vi "SLL DE AO Driver.vi"(6 "AO Channel Value Array":dbl[](array[numeric]), 7 "AO Driver Option":T2=enum."Read Full Status", 8 "error in (no error)":errorcluster, 9 "AO Channel Value":dbl, 10 "AO Channel Name Array":T1[](array[typedef]), 11 "AO Channel Name":T1) -> (0 "error out":errorcluster)   [LabVIEW 2013]
doc: "Copyright © 2005, Soliton Technologies.\nAll rights reserved."
uses:
  Controls/SLL DE AO Global Options.ctl
  Controls/SLL DE List of Analog Outputs.ctl
  Controls/SLL DE DAQ Global Options.ctl
  Controls/SLL DE DAQ Global Elements.ctl
  Controls/SLL DE AO Min Max Range Checking Options.ctl
  Controls/SLL DE AO Safe Value Global Options.ctl
  <vilib>/DAQmx/write.llb/DAQmx Write (Analog DBL 1Chan 1Samp).vi
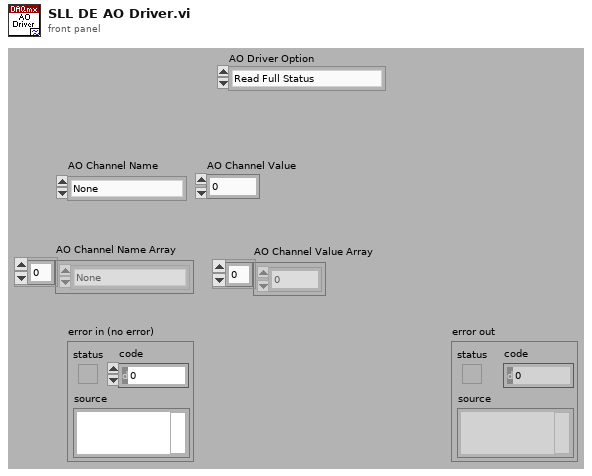
[diagram p1: front panel]
types:
  T1 = typedef "SLL DE List of Analog Outputs.ctl" = enum16{"None"}
  T2 = typedef "SLL DE AO Global Options.ctl" = enum16{"Init", "Write Line", "Write Array", "Read Line", "Read Array", "Read Full Status", "Restart AO", "Send to Safe Mode", "Stop AO"}
  T3 = typedef "SLL DE DAQ Global Elements.ctl" = enum16{"AI Error", "AO Error", "DI Error", "DO Error", "AI Restart", "DI Restart", "AI Running", "AO Running", "DI Running", "DO Running", "DAQ Exit?"}
  T4 = typedef "SLL DE DAQ Global Options.ctl" = enum16{"Init", "Write 1", "Read 1", "Write Array", "Read Array", "Clear"}
  T5 = typedef "SLL DE AO Min Max Range Checking Options.ctl" = enum16{"Initalize Channel Range", "Check Single AO Channel", "Check Multiple AO Channels"}
  T6 = typedef "SLL DE AO Safe Value Global Options.ctl" = enum16{"Read", "Write"}
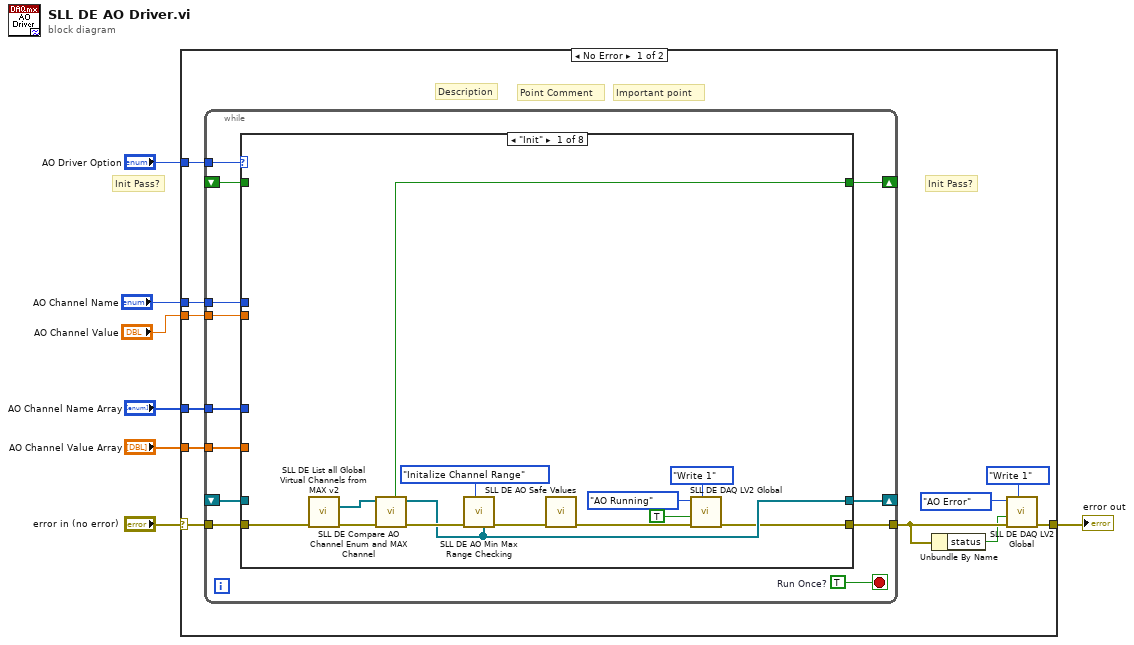
[diagram p0: block diagram]
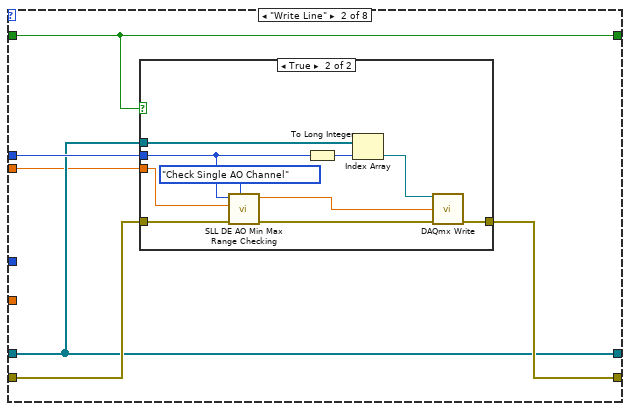
[diagram p2: hidden frame]
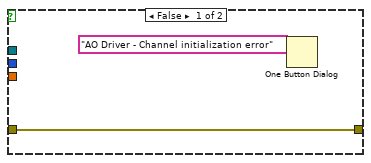
[diagram p3: hidden frame]
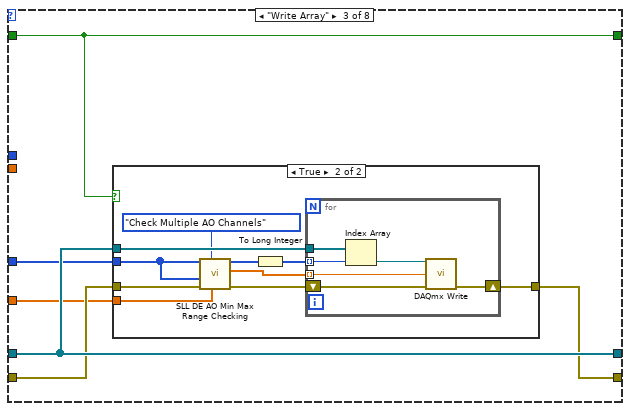
[diagram p4: hidden frame]
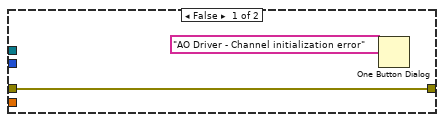
[diagram p5: hidden frame]
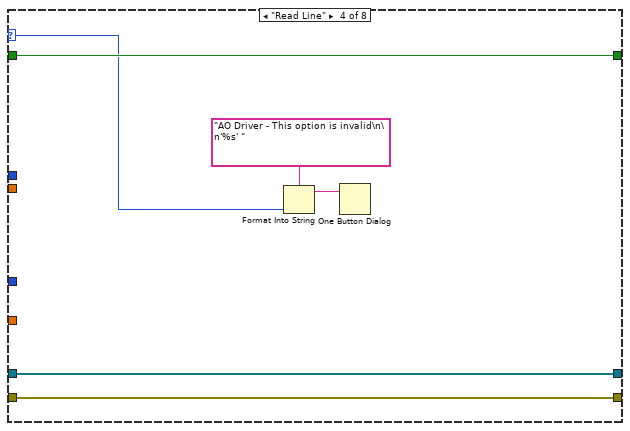
[diagram p6: hidden frame]
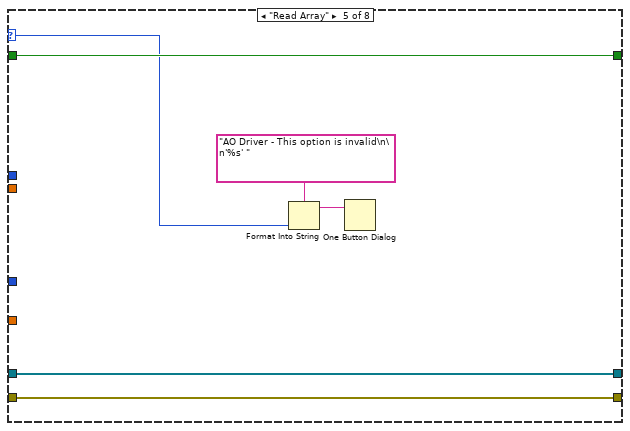
[diagram p7: hidden frame]
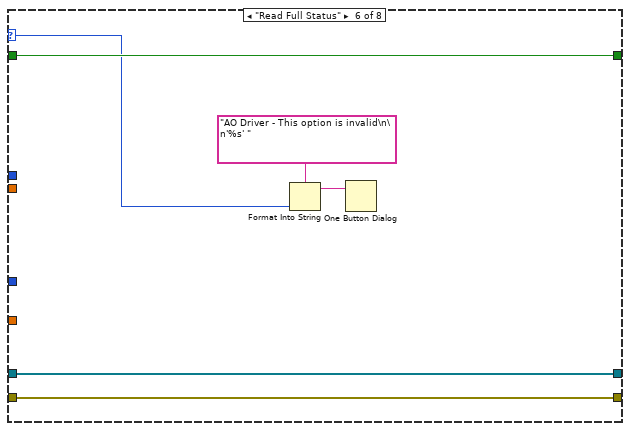
[diagram p8: hidden frame]
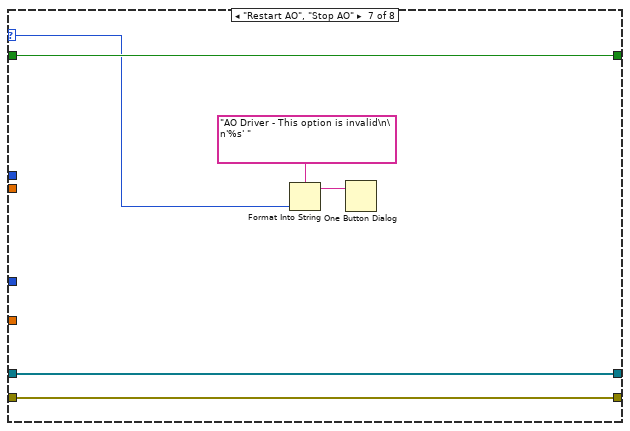
[diagram p9: hidden frame]
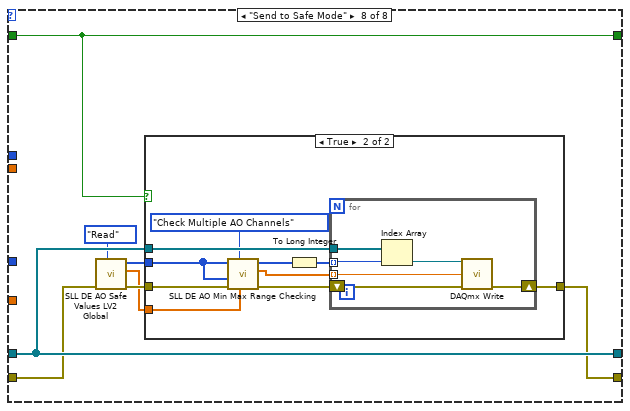
[diagram p10: hidden frame]
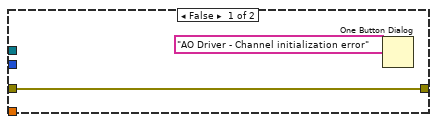
[diagram p11: hidden frame]
diagram:
  # "Init Pass?"
  n1 = case shown="No Error" "error in (no error)" {
    selector: "error in (no error)" -> [w18 w134]
    tunnel: [w10 w134] -> w6
    tunnel: "AO Driver Option" -> [w17 _]
    tunnel: "AO Channel Name" -> [w16 _]
    tunnel: "AO Channel Name Array" -> [w15 _]
    tunnel: "AO Channel Value" -> [w14 _]
    tunnel: "AO Channel Value Array" -> [w13 _]
    frame No Error {
      # "Init Pass?"
      # "Point Comment"
      # "Important point"
      # "Description"
      n2 = while {
        tunnel: w18 -> [w29]
        tunnel: [w28] -> w9
        shift-right: [w27] -> _
        shift-left: _ -> [w24]
        shift-right: [w26] -> _
        shift-left: _ -> [w23]
        tunnel: w17 -> [w25]
        tunnel: w16 -> [w22]
        tunnel: w15 -> [w21]
        tunnel: w14 -> [w20]
        tunnel: w13 -> [w19]
        stop <- w30 stop-if-true
        w30 = TRUE  # Run Once?
        n3 = case shown="\"Init\"" w25 {
          selector: w25 -> [_ _ _ w85 w91 w97 w103 _]
          tunnel: w29 -> [w41 w49 w66 w88 w94 w100 w106 w112]
          tunnel: [w31 w48 w65 w88 w94 w100 w106 w114] -> w28
          tunnel: [w40 w44 w64 w89 w96 w102 w108 w115] -> w27
          tunnel: [w37 w46 w67 w90 w95 w101 w107 w116] -> w26
          tunnel: w24 -> [_ w44 w64 w89 w96 w102 w108 w115]
          tunnel: w23 -> [_ w46 w67 w90 w95 w101 w107 w116]
          tunnel: w22 -> [_ w47 _ _ _ _ _ _]
          tunnel: w21 -> [_ _ w63 _ _ _ _ _]
          tunnel: w20 -> [_ w45 _ _ _ _ _ _]
          tunnel: w19 -> [_ _ w62 _ _ _ _ _]
          frame "Init" {
            n4 = call "SLL DE List all Global Virtual Channels from MAX v2.vi"("error in (no error)"=w41) -> ("error out"=w43:errorcluster, "Analog Output"=w42:refnum<k21>[])  [unwired: 4 in, 5 out]
            n5 = call "SLL DE Compare AO Channel Enum and MAX Channel.vi"("error in (no error)"=w43, "Analog Output Channels"=w42) -> ("error out"=w38:errorcluster, "Channels Out"=w37:refnum<k21>[], "Pass?"=w40:bool)  [unwired: 7 in]
            n6 = call "SLL DE AO Min Max Range Checking.vi"("Analog Output Channels"=w37, "Option"=SLL_DE_AO_Min_Max_Range_Checking_Options."Initalize Channel Range", "error in (no error)"=w38) -> ("error out"=w36:errorcluster)  [unwired: 6 in, 2 out]
            n7 = call "SLL DE AO Safe Values.vi"("error in (no error)"=w36) -> ("error out"=w32:errorcluster)  [unwired: 8 in, 2 out]
            n8 = call "SLL DE DAQ LV2 Global.vi"("Option"=SLL_DE_DAQ_Global_Options."Write 1", "error in (no error)"=w32, "Status In"=TRUE, "Element"=SLL_DE_DAQ_Global_Elements."AO Running") -> ("error out"=w31:errorcluster)  [unwired: 5 in, 2 out]
          }
          frame "Write Line" {
            n9 = case shown="True" w44 {
              tunnel: w49 -> [w51 w56]
              tunnel: [w51 w61] -> w48
              tunnel: w47 -> [_ w54]
              tunnel: w46 -> [_ w60]
              tunnel: w45 -> [_ w53]
              frame False {
                n10 = One Button Dialog(message="AO Driver - Channel initialization error") -> ()  [unwired: 1 in, 1 out]
              }
              frame True {
                n11 = call "SLL DE AO Min Max Range Checking.vi"("Option"=SLL_DE_AO_Min_Max_Range_Checking_Options."Check Single AO Channel", "error in (no error)"=w56, "AO Value"=w53, "AO Channel Name"=w54) -> ("error out"=w55:errorcluster, "AO Value Out"=w52:dbl)  [unwired: 5 in, 1 out]
                n12 = To Long Integer(number=w54) -> (32bit integer=w58:i32)
                n13 = Index Array(array=w60, index=w58) -> (element=w59:refnum<k21>)
                n14 = call-poly <vilib>:"DAQmx Write.vi"("task/channels in"=w59, "data"=w52, "error in"=w55) -> ("error out"=w61:errorcluster)  [unwired: 10 in, 2 out]
              }
            }
          }
          frame "Write Array" {
            n15 = case shown="True" w64 {
              tunnel: w66 -> [w69 w73]
              tunnel: [w69 w78] -> w65
              tunnel: w63 -> [_ w74]
              tunnel: w67 -> [_ w77]
              tunnel: w62 -> [_ w72]
              frame False {
                n16 = One Button Dialog(message="AO Driver - Channel initialization error") -> ()  [unwired: 1 in, 1 out]
              }
              frame True {
                n17 = call "SLL DE AO Min Max Range Checking.vi"("AO Values In"=w72, "Option"=SLL_DE_AO_Min_Max_Range_Checking_Options."Check Multiple AO Channels", "error in (no error)"=w73, "AO Channels Name"=w74) -> ("error out"=w70:errorcluster, "AO Values Out"=w71:dbl[])  [unwired: 5 in, 1 out]
                n18 = To Long Integer(number=w74) -> (32bit integer=w76:i32[])
                n19 = for {
                  tunnel: w76 -> [w82] mode=indexing
                  tunnel: w77 -> [w81]
                  tunnel: w71 -> [w79] mode=indexing
                  shift-right: [w83] -> w78
                  shift-left: w70 -> [w84]
                  n20 = Index Array(array=w81, index=w82) -> (element=w80:refnum<k21>)
                  n21 = call-poly <vilib>:"DAQmx Write.vi"("task/channels in"=w80, "data"=w79, "error in"=w84) -> ("error out"=w83:errorcluster)  [unwired: 10 in, 2 out]
                }
              }
            }
          }
          frame "Read Line" {
            n22 = Format Into String(format string="AO Driver - This option is invalid\n\n'%s' " ("message"), w85) -> (resulting string=w86:string)  [unwired: 2 in, 1 out]
            n23 = One Button Dialog(message=w86) -> ()  [unwired: 1 in, 1 out]
          }
          frame "Read Array" {
            n24 = Format Into String(format string="AO Driver - This option is invalid\n\n'%s' " ("message"), w91) -> (resulting string=w92:string)  [unwired: 2 in, 1 out]
            n25 = One Button Dialog(message=w92) -> ()  [unwired: 1 in, 1 out]
          }
          frame "Read Full Status" {
            n26 = Format Into String(format string="AO Driver - This option is invalid\n\n'%s' " ("message"), w97) -> (resulting string=w98:string)  [unwired: 2 in, 1 out]
            n27 = One Button Dialog(message=w98) -> ()  [unwired: 1 in, 1 out]
          }
          frame "Restart AO", "Stop AO" {
            n28 = Format Into String(format string="AO Driver - This option is invalid\n\n'%s' " ("message"), w103) -> (resulting string=w104:string)  [unwired: 2 in, 1 out]
            n29 = One Button Dialog(message=w104) -> ()  [unwired: 1 in, 1 out]
          }
          frame "Send to Safe Mode" {
            n30 = call "SLL DE AO Safe Values LV2 Global.vi"("Cases"=SLL_DE_AO_Safe_Value_Global_Options."Read", "error in (no error)"=w112) -> ("error out"=w111:errorcluster, "Value Array Out"=w110:dbl[], "Elements Out"=w109:T1[])  [unwired: 7 in]
            n31 = case shown="True" w115 {
              tunnel: w111 -> [w118 w123]
              tunnel: [w118 w127] -> w114
              tunnel: w109 -> [_ w122]
              tunnel: w116 -> [_ w126]
              tunnel: w110 -> [_ w120]
              frame False {
                n32 = One Button Dialog(message="AO Driver - Channel initialization error") -> ()  [unwired: 1 in, 1 out]
              }
              frame True {
                n33 = call "SLL DE AO Min Max Range Checking.vi"("AO Values In"=w120, "Option"=SLL_DE_AO_Min_Max_Range_Checking_Options."Check Multiple AO Channels", "error in (no error)"=w123, "AO Channels Name"=w122) -> ("error out"=w121:errorcluster, "AO Values Out"=w119:dbl[])  [unwired: 5 in, 1 out]
                n34 = To Long Integer(number=w122) -> (32bit integer=w125:i32[])
                n35 = for {
                  tunnel: w125 -> [w131] mode=indexing
                  tunnel: w126 -> [w130]
                  tunnel: w119 -> [w128] mode=indexing
                  shift-right: [w132] -> w127
                  shift-left: w121 -> [w133]
                  n36 = Index Array(array=w130, index=w131) -> (element=w129:refnum<k21>)
                  n37 = call-poly <vilib>:"DAQmx Write.vi"("task/channels in"=w129, "data"=w128, "error in"=w133) -> ("error out"=w132:errorcluster)  [unwired: 10 in, 2 out]
                }
              }
            }
          }
        }
      }
      n38 = Unbundle By Name(w9) -> ("status"=w8:bool)
      n39 = call "SLL DE DAQ LV2 Global.vi"("Option"=SLL_DE_DAQ_Global_Options."Write 1", "error in (no error)"=w9, "Status In"=w8, "Element"=SLL_DE_DAQ_Global_Elements."AO Error") -> ("error out"=w10:errorcluster)  [unwired: 5 in, 2 out]
    }
    frame Error {
    }
  }
  "error out" <- w6
